vi "Path Separator.vi"() -> (3 "separator":string)   [LabVIEW 2014, in "lvprj2html.lvlib"]
uses:
  lvprj2html.lvlib
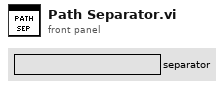
[diagram p1: front panel]
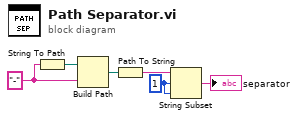
[diagram p0: block diagram]
diagram:
  w2 = 1 ("offset (0)")
  w6 = "-" ("name or relative path")
  n1 = String To Path(string=w6) -> (path=w5:path)
  n2 = Build Path(base path=w5, name or relative path=w6) -> (appended path=w4:path)
  n3 = Path To String(path=w4) -> (string=w3:string)
  n4 = String Subset(string=w3, offset (0)=w2, length (rest)=w2) -> (substring=→"separator":string)
